vi "addError.vi"(7 "execution time (sec)":dbl, 8 "error in (no error)":errorcluster, 9 "test error":errorcluster, 10 "test":refnum<class>, 11 "TestTestResult in":refnum<class "_TextTestResult.JUnitXML.lvclass">) -> (0 "error out":errorcluster, 3 "TestTestResult out":refnum<class "_TextTestResult.JUnitXML.lvclass">)   [LabVIEW 2013, in "_TextTestResult.JUnitXML.lvclass"]
uses:
  _TextTestResult.JUnitXML.lvclass
  <vilib>/addons/_JKI Toolkits/VI Tester/_TextTestResult.llb/_TextTestResult.lvclass
  <vilib>/addons/_JKI Toolkits/VI Tester/TestResult.llb/resultStatus--enum.ctl
  <vilib>/addons/_JKI Toolkits/VI Tester/TestResult.llb/TestResult.lvclass
panel:
  # "JKI VI Tester for LabVIEW\nhttp://jkisoft.com/vi-tester\nCopyright (C) 2007-2009, JKI <info@jkisoft.com>\nALL RIGHTS RESERVED"
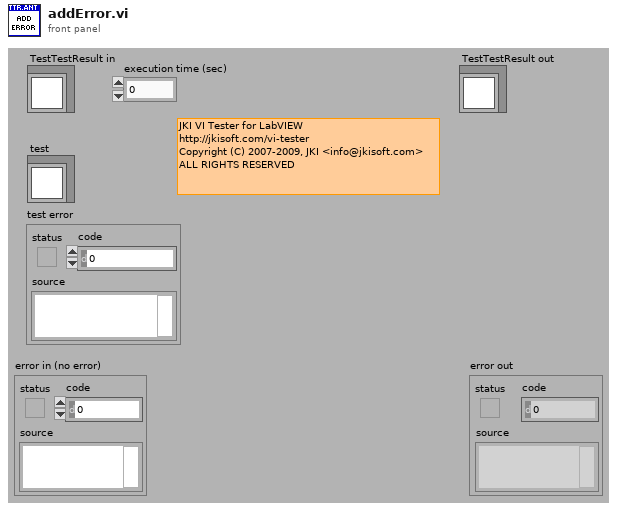
[diagram p1: front panel]
types:
  T1 = typedef "TestResult.lvclass/resultStatus--enum.ctl" = enum16{"testPass", "testFailure", "testError", "testSkipped"}
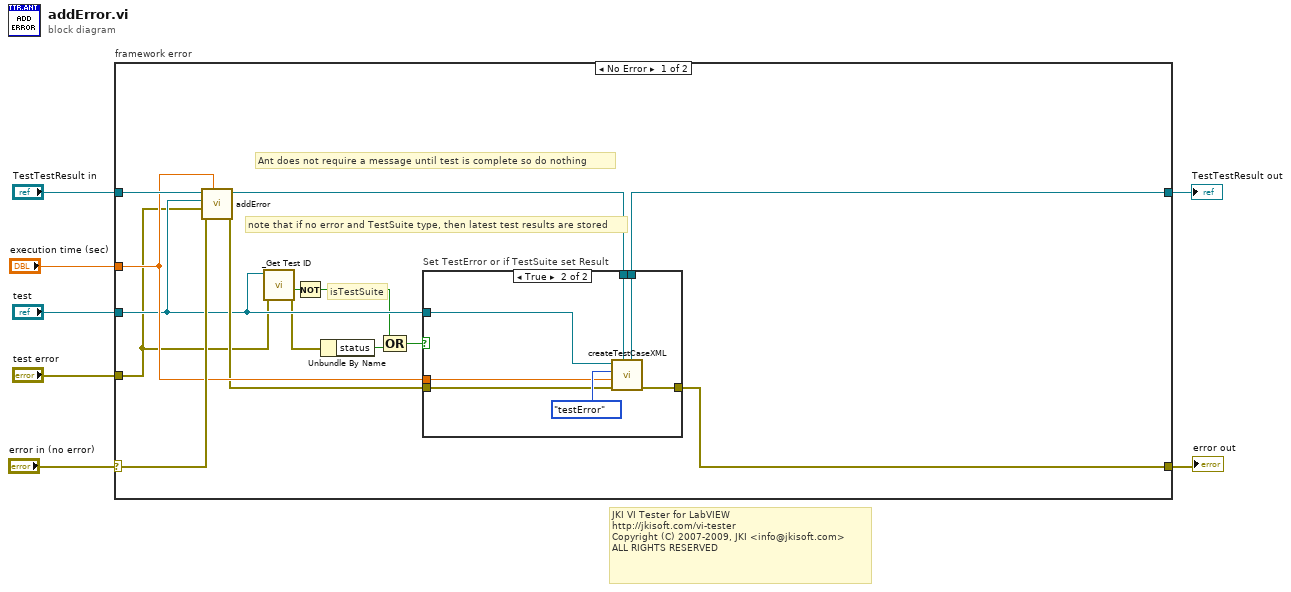
[diagram p0: block diagram]
diagram:
  # "JKI VI Tester for LabVIEW\nhttp://jkisoft.com/vi-tester\nCopyright (C) 2007-2009, JKI <info@jkisoft.com>\nALL RIGHTS RESERVED"
  n1 = case "framework error" shown="No Error" "error in (no error)" {
    selector: "error in (no error)" -> [w20 w32]
    tunnel: [w18 w32] -> w6
    tunnel: [w8 w31] -> w4
    tunnel: "TestTestResult in" -> [w21 w31]
    tunnel: "test error" -> [w14 _]
    tunnel: "test" -> [w16 _]
    tunnel: "execution time (sec)" -> [w19 _]
    frame No Error {
      # "note that if no error and TestSuite type, then latest test results are stored"
      # "isTestSuite"
      # "Ant does not require a message until test is complete so do nothing"
      n2 = call-parent "addError.vi"("execution time (sec)"=w19, "error in (no error)"=w20, "test error"=w14, "test"=w16, "TestTestResult in"=w21) -> ("error out"=w17:errorcluster, "TestTestResult out"=w9:refnum<class "_TextTestResult.JUnitXML.lvclass">)  [unwired: 5 in]
      n3 = call "_Get Test ID.vi"("error in"=w14, "Test In"=w16) -> ("error out"=w11:errorcluster, "IsTestCase"=w13:bool)  [unwired: 5 in, 3 out]
      n4 = Not(x=w13) -> (.not. x?=w12:bool)
      n5 = Unbundle By Name(w11) -> ("status"=w15:bool)
      n6 = Compound Arithmetic op=OR(w12, w15) -> (w10:bool)
      n7 = case "Set TestError or if TestSuite set Result" shown="True" w10 {
        tunnel: w17 -> [w23 w29]
        tunnel: w19 -> [_ w28]
        tunnel: w16 -> [_ w27]
        tunnel: w9 -> [w22 w26]
        tunnel: [w23 w25] -> w18
        tunnel: [w22 w24] -> w8
        frame False {
        }
        frame True {
          n8 = call "createTestCaseXML.vi"("TestTestResult.Ant"=w26, "error in (no error)"=w29, "execution time (sec)"=w28, "resultStatus"=resultStatus--enum."testError", "Test Out"=w27) -> ("error out"=w25:errorcluster, "TestTestResult.Ant Out"=w24:refnum<class "_TextTestResult.JUnitXML.lvclass">)  [unwired: 5 in]
        }
      }
    }
    frame Error {
    }
  }
  "error out" <- w6
  "TestTestResult out" <- w4
